vi "顺序打印我要自学网.vi"() -> ()   [LabVIEW 2018]
panel:
  out "字符串":string
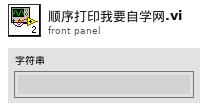
[diagram p1: front panel]
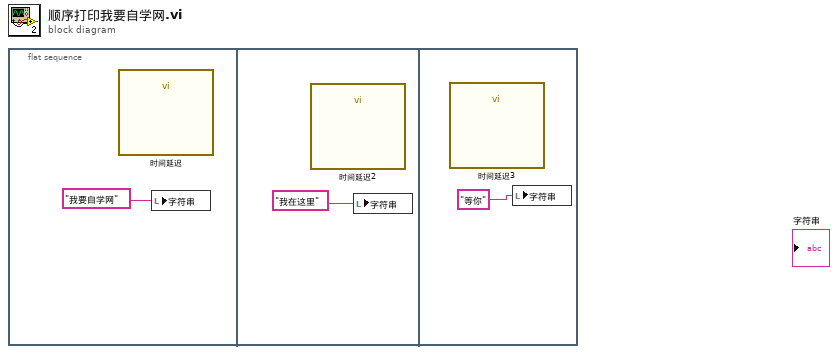
[diagram p0: block diagram]
diagram:
  n1 = flat-sequence {
    frame #0 {
      n2 = call "时间延迟"() -> ()  [unwired: 11 in, 1 out]
      n3 = local write "字符串"("我要自学网") -> ()
    }
    frame #1 {
      n4 = call "时间延迟2"() -> ()  [unwired: 11 in, 1 out]
      n5 = local write "字符串"("我在这里") -> ()
    }
    frame #2 {
      n6 = call "时间延迟3"() -> ()  [unwired: 11 in, 1 out]
      n7 = local write "字符串"("等你") -> ()
    }
  }
